vi "RSZVB Get Source Power Calibration Converter State.vi"(8 "error in (no error)":errorcluster {"code" format="%.0x"}, 9 "Converter (1)":i32=1, 10 "Channel (1)":i32=1, 11 "VISA session":refnum<visa-resource-name>) -> (0 "error out":errorcluster {"code" format="%.0x"}, 2 "Calibration Converter":bool, 3 "dup VISA session":refnum<visa-resource-name>)   [LabVIEW 2011]
doc: "This VI returns the source power calibration for channel <Ch> and for an external frequency converter number <Con> state. \n\nRemote-control command(s):\nSOURce<Ch>:POWer<Pt>:CORRection:CONVerter<Con>[:STATe]?"
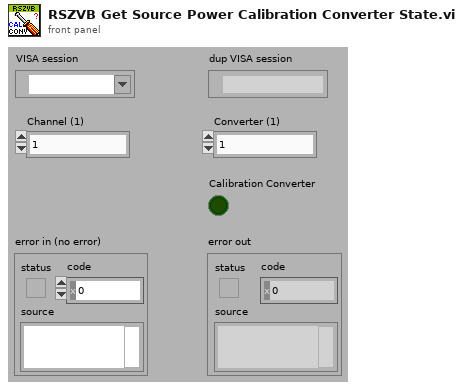
[diagram p1: front panel]
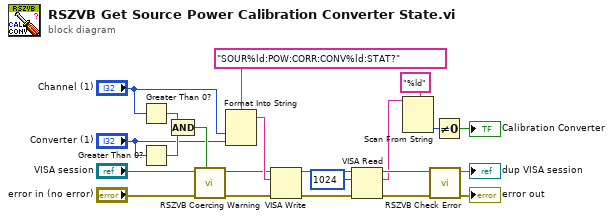
[diagram p0: block diagram]
diagram:
  n1 = Greater Than 0?(x="Channel (1)") -> (x > 0?=w18:bool)
  n2 = Greater Than 0?(x="Converter (1)") -> (x > 0?=w17:bool)
  n3 = Compound Arithmetic op=AND(w18, w17) -> (w16:bool)
  n4 = call "RSZVB Coercing Warning.vi"("In Range?"=w16, "error in (no error)"="error in (no error)", "VISA session"="VISA session") -> ("error out"=w21:errorcluster, "dup VISA session"=w20:refnum<visa-resource-name>)  [unwired: 7 in]
  n5 = Format Into String(format string="SOUR%ld:POW:CORR:CONV%ld:STAT?", "Channel (1)", "Converter (1)") -> (resulting string=w22:string)  [unwired: 2 in, 1 out]
  n6 = VISA Write(VISA resource name=w20, write buffer=w22, error in (no error)=w21) -> (VISA resource name out=w11:refnum<visa-resource-name>, error out=w12:errorcluster)  [unwired: 1 out]
  n7 = VISA Read(VISA resource name=w11, byte count=u32 1024, error in (no error)=w12) -> (VISA resource name out=w13:refnum<visa-resource-name>, read buffer=w2:string, error out=w14:errorcluster)  [unwired: 1 out]
  n8 = Scan From String(format string="%ld", input string=w2) -> (output 1=w3:i32)  [unwired: 3 in, 3 out]
  n9 = call "RSZVB Check Error.vi"("error in (no error)"=w14, "VISA session"=w13) -> ("error out"=→"error out":errorcluster, "dup VISA session"=→"dup VISA session":refnum<visa-resource-name>)  [unwired: 8 in]
  n10 = Not Equal To 0?(x=w3) -> (x != 0?=→"Calibration Converter":bool)
